vi "openbci_config_channels.vi"(1 "SRB1_SET? (F)":bool, 4 "SRB2_SET? (T)":bool=TRUE, 5 "ADC_channel_input_soruce":T1, 6 "BIAS_SET? (T)":bool=TRUE, 7 "Gain_ADS1299":T2=enum."24x", 8 "error in (no error)":errorcluster, 9 "channel":T5, 10 "on? (T)":bool=TRUE, 11 "OBCI dev in":T3={"COM port"="", "n_ch (8)"=enum."8 Channels", "delay_tx"=50}) -> (0 "error out":errorcluster, 3 "OBCI dev out":T3={"COM port"="", "n_ch (8)"=enum."8 Channels", "delay_tx"=50})   [LabVIEW 2013]
doc: "Send the configuration for a specific channel (1 - 16)"
uses:
  Control Def/channels_enum.ctl
  Control Def/openbci_device.ctl
  Control Def/channel_count.ctl
  Control Def/gain_ADS1299.ctl
  Control Def/acd_input_source.ctl
  Control Def/string_channel_id.ctl
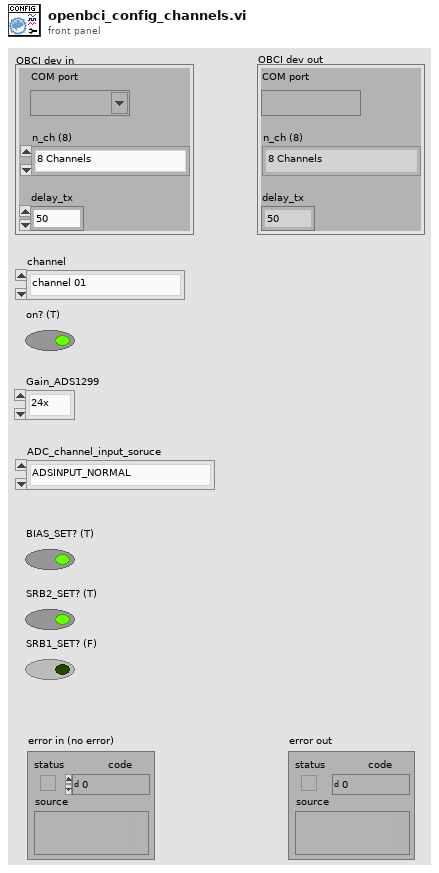
[diagram p1: front panel]
types:
  T1 = typedef "acd_input_source.ctl" = enum16{"ADSINPUT_NORMAL", "ADSINPUT_SHORTED", "ADSINPUT_BIAS_MEAS", "ADSINPUT_MVDD", "ADSINPUT_TEMP", "ADSINPUT_TESTING", "ADSINPUT_BIAS_DRP", "ADSINPUT_BIAS_DRN"}
  T2 = typedef "gain_ADS1299.ctl" = enum16{"1x", "2x", "4x", "8x", "16x", "24x"}
  T3 = typedef "openbci_device.ctl" = cluster{"COM port":refnum<visa-resource-name>, "n_ch (8)":T4, "delay_tx":u32}
  T4 = typedef "channel_count.ctl" = enum16{"8 Channels", "16 Channels"}
  T5 = typedef "channels_enum.ctl" = enum16{"channel 01", "channel 02", "channel 03", "channel 04", "channel 05", "channel 06", "channel 07", "channel 08", "Channel 09", "Channel 10", "Channel 11", "Channel 12", "Channel 13", "Channel 14", "Channel 15", "Channel 16"}
  T6 = typedef "string_channel_id.ctl" = string[]
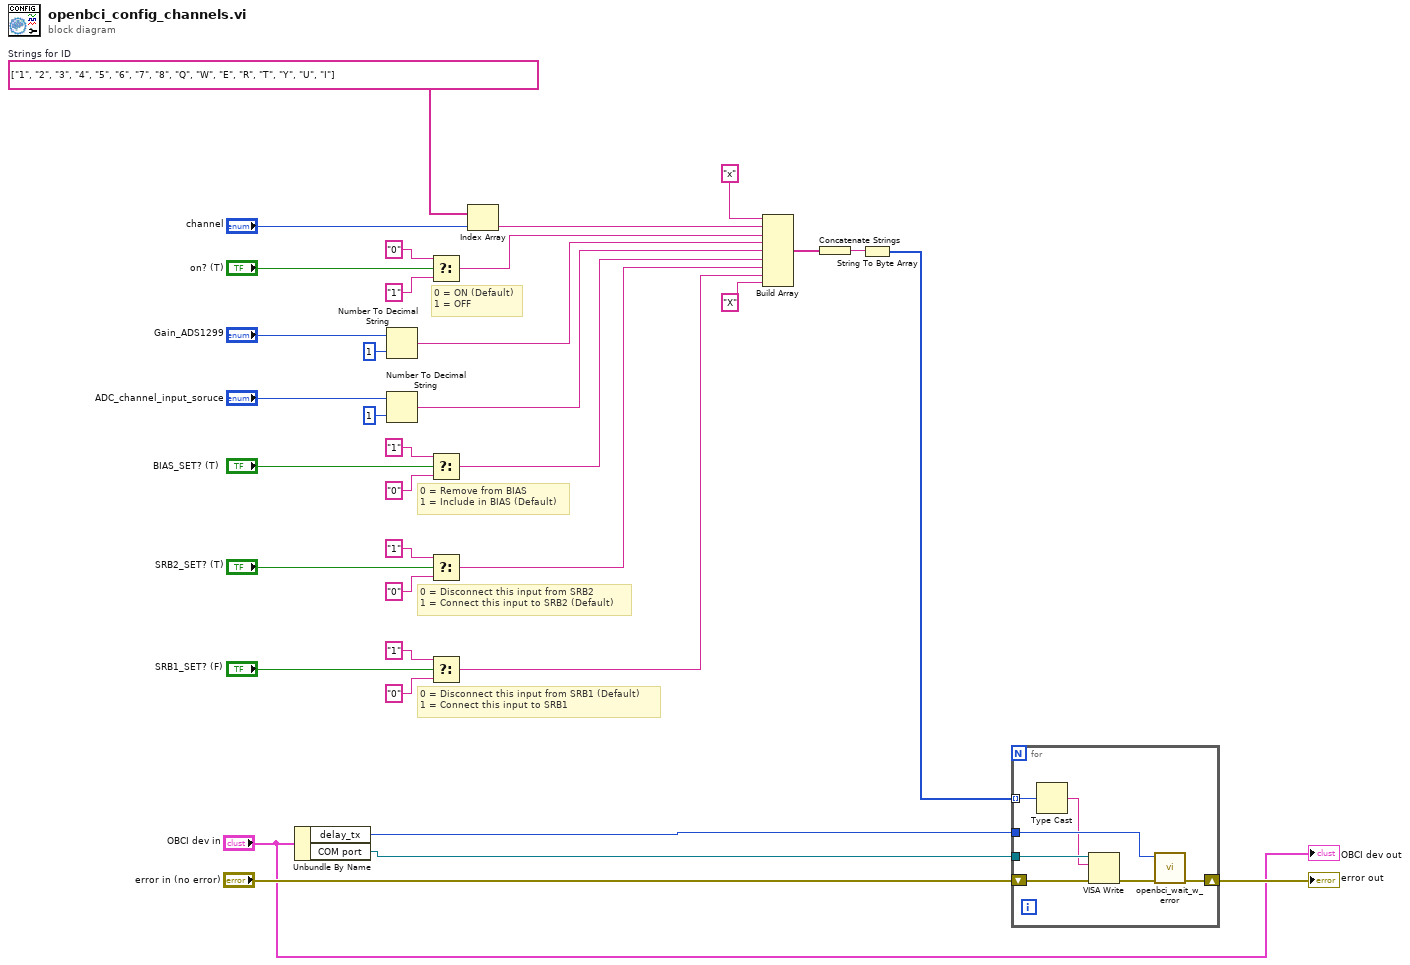
[diagram p0: block diagram]
diagram:
  w29 = T6 ["1", "2", "3", "4", "5", "6", "7", "8", "Q", "W", "E", "R", "T", "Y", "U", "I"]  # Strings for ID
  # "0 = Disconnect this input from SRB1 (Default)\n1 = Connect this input to SRB1"
  # "0 = Disconnect this input from SRB2\n1 = Connect this input to SRB2 (Default)"
  # "0 = Remove from BIAS\n1 = Include in BIAS (Default)"
  # "0 = ON (Default)\n1 = OFF"
  n1 = Unbundle By Name("OBCI dev in") -> ("delay_tx"=w31:u32, "COM port"=w33:refnum<visa-resource-name>)
  n2 = Number To Decimal String(number="Gain_ADS1299", width (-)=i16 1) -> (decimal integer string=w21:string)
  n3 = Number To Decimal String(number="ADC_channel_input_soruce", width (-)=i16 1) -> (decimal integer string=w18:string)
  n4 = Select(t="0" ("element"), s="on? (T)", f="1" ("element")) -> (s? t:f=w24:string)
  n5 = Select(t="1" ("element"), s="BIAS_SET? (T)", f="0" ("element")) -> (s? t:f=w8:string)
  n6 = Select(t="1" ("element"), s="SRB2_SET? (T)", f="0" ("element")) -> (s? t:f=w7:string)
  n7 = Select(t="1" ("element"), s="SRB1_SET? (F)", f="0" ("element")) -> (s? t:f=w6:string)
  n8 = Index Array(array=w29, index="channel") -> (element=w28:string)
  n9 = Build Array("x" ("element"), w28, w24, w21, w18, w8, w7, w6, "X" ("element")) -> (w3:string[])
  n10 = Concatenate Strings(w3) -> (w2:string)
  n11 = String To Byte Array(string=w2) -> (unsigned byte array=w1:u8[])
  n12 = for {
    tunnel: w33 -> [w41]
    tunnel: w31 -> [w38]
    tunnel: w1 -> [w36] mode=indexing
    shift-right: [w39] -> w32
    shift-left: "error in (no error)" -> [w42]
    n13 = Type Cast(x=w36) -> (*(type *) &x=w37:string)  [unwired: 1 in]
    n14 = VISA Write(VISA resource name=w41, write buffer=w37, error in (no error)=w42) -> (error out=w40:errorcluster)  [unwired: 2 out]
    n15 = call "openbci_wait_w_error.vi"("error in (no error)"=w40, "milliseconds to wait"=w38) -> ("error out"=w39:errorcluster)  [unwired: 9 in]
  }
  "error out" <- w32
  "OBCI dev out" <- "OBCI dev in"
